vi "slope corrector.vi"(8 "Pump Calibration":T1, 11 "flow rate":dbl[unit]) -> (3 "modified flow rate":dbl[unit])   [LabVIEW 2012]
uses:
  calibration values.ctl
  <vilib>/Analysis/NI_AALPro.lvlib
panel:
  out "error":i32
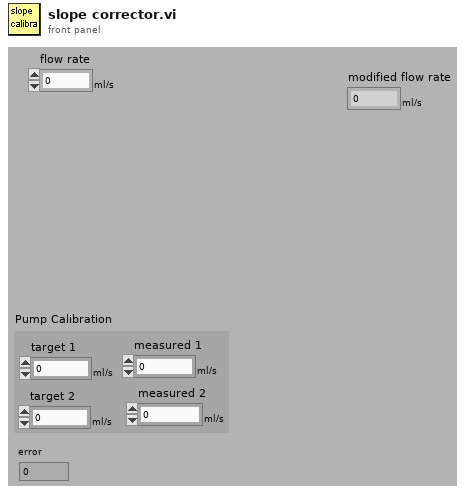
[diagram p1: front panel]
types:
  T1 = typedef "calibration values.ctl" = cluster{"target 1":dbl[unit], "target 2":dbl[unit], "measured 1":dbl[unit], "measured 2":dbl[unit]}
  T2 = cluster{"target 1":dbl, "target 2":dbl, "measured 1":dbl, "measured 2":dbl}
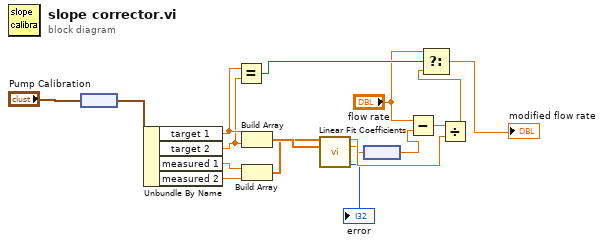
[diagram p0: block diagram]
diagram:
  n1 = node("Pump Calibration") -> (w12:T2)
  n2 = Unbundle By Name(w12) -> ("target 1"=w6:dbl, "target 2"=w5:dbl, "measured 1"=w16:dbl, "measured 2"=w15:dbl)
  n3 = Equal?(x=w6, y=w5) -> (x = y?=w4:bool)
  n4 = Build Array(w6, w5) -> (w14:dbl[])
  n5 = Build Array(w16, w15) -> (w13:dbl[])
  n6 = call <vilib>:"Linear Fit Coefficients.vi"("Y"=w13, "X"=w14) -> ("slope"=w9:dbl, "intercept"=w8:dbl, "error"=→"error":i32)  [unwired: 11 in]
  n7 = node(w8) -> (w11:dbl[unit])
  n8 = Subtract(x="flow rate", y=w11) -> (x-y=w10:dbl[unit])
  n9 = Divide(x=w10, y=w9) -> (x/y=w2:dbl[unit])
  n10 = Select(t="flow rate", s=w4, f=w2) -> (s? t:f=→"modified flow rate":dbl[unit])
